vi "Increment Job Count.vi"(8 "error in (no error)":errorcluster, 11 "Worker In":refnum<class "Worker.lvclass">) -> (0 "error out":errorcluster, 3 "Worker Out":refnum<class "Worker.lvclass">)   [LabVIEW 2020, in "Worker.lvclass"]
uses:
  Worker.lvclass
  Worker.lvclass/Worker.ctl
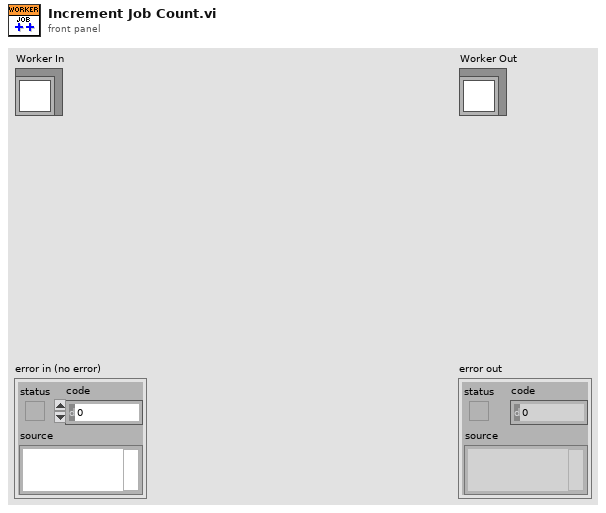
[diagram p1: front panel]
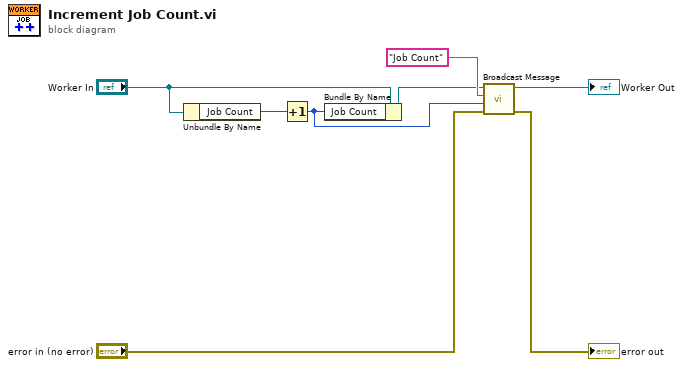
[diagram p0: block diagram]
diagram:
  n1 = Unbundle By Name("Worker In") -> ("Job Count"=w2:u32)
  n2 = Increment(x=w2) -> (x+1=w1:u32)
  n3 = Bundle By Name(cluster="Worker In", "Job Count"=w1) -> (w3:refnum<class "Worker.lvclass">)
  n4 = call-dynamic "Broadcast Message.vi"("error in (no error)"="error in (no error)", "Message Data"=w1, "Message"="Job Count", "Rig Process In"=w3) -> ("error out"=→"error out":errorcluster, "Rig Process Out"=→"Worker Out":refnum<class "Worker.lvclass">)  [unwired: 6 in]
